vi "ni579x Validate LO Frequency.vi"(0 "Register Bus":refnum<class "ni579x Register Bus v1 Host.lvclass">=refnum, 1 "scope":string, 5 "frequency [Hz]":dbl format="%#_6p", 11 "Error In":errorcluster) -> (4 "Register Bus (out)":refnum<class "ni579x Register Bus v1 Host.lvclass">, 6 "coerced frequency [Hz]":dbl format="%#_6p", 15 "Error Out":errorcluster)   [LabVIEW 2015]
uses:
  <instrlib>/ni579x/Register Bus/v1/Host/ni579x Register Bus v1 Host.lvclass
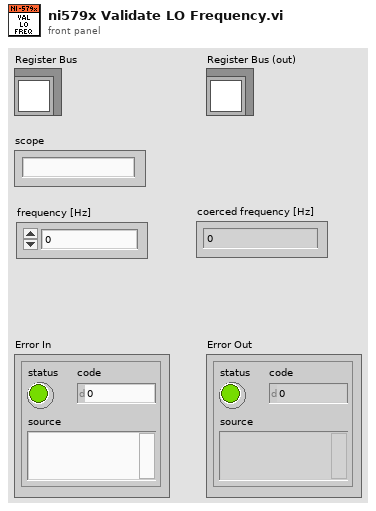
[diagram p1: front panel]
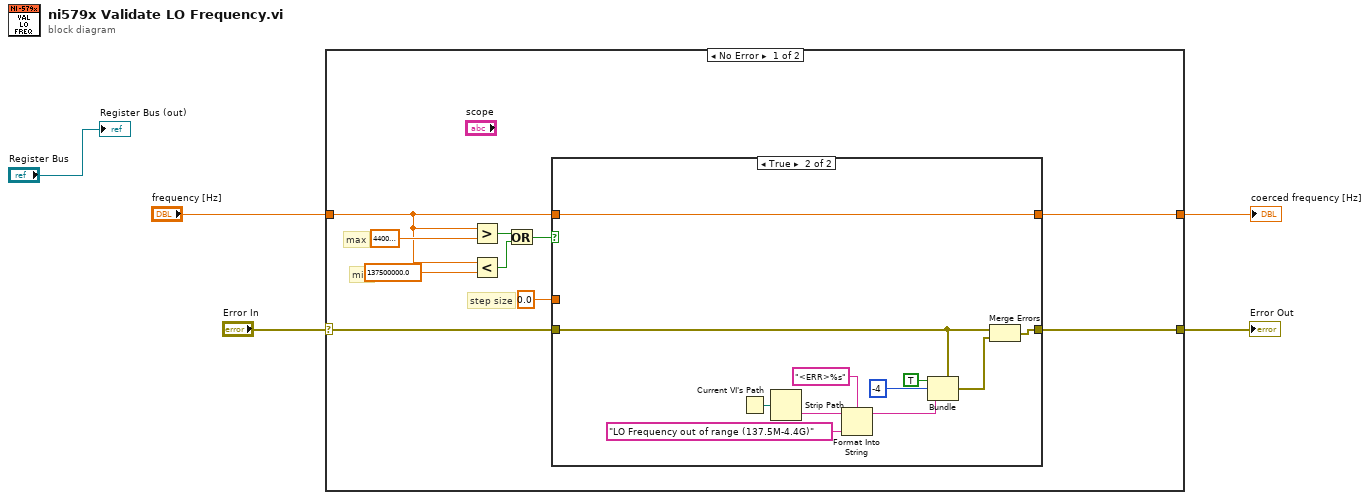
[diagram p0: block diagram]
diagram:
  n1 = case shown="No Error" "Error In" {
    selector: "Error In" -> [w8 w30]
    tunnel: [w6 w30] -> w4
    tunnel: "frequency [Hz]" -> [w10 w29]
    tunnel: [w7 w29] -> w1
    frame No Error {
      # "min"
      # "max"
      # "step size"
      n2 = Greater?(x=w10, y=4400000000.0) -> (0:w13:bool)
      n3 = Less?(x=w10, y=137500000.0) -> (x < y?=w12:bool)
      n4 = Or(x=w13, y=w12) -> (x .or. y?=w11:bool)
      n5 = case shown="True" w11 {
        tunnel: w10 -> [w16 w21]
        tunnel: 0.0 -> [_ _]
        tunnel: [w16 w21] -> w7
        tunnel: w8 -> [w17 w24]
        tunnel: [w17 w22] -> w6
        frame False {
        }
        frame True {
          n6 = Current VI's Path() -> (path=w27:path)
          n7 = Strip Path(path=w27) -> (name=w26:string)  [unwired: 1 out]
          n8 = Format Into String(format string="<ERR>%s", initial string=w26, "LO Frequency out of range (137.5M-4.4G)" ("input 1")) -> (resulting string=w25:string)  [unwired: 1 in, 1 out]
          n9 = Bundle(cluster=w24, "status"=TRUE, "code"=-4, "source"=w25) -> (w23:errorcluster)
          n10 = Merge Errors(w24, w23) -> (w22:errorcluster)
        }
      }
    }
    frame Error {
    }
  }
  "Error Out" <- w4
  "coerced frequency [Hz]" <- w1
  "Register Bus (out)" <- "Register Bus"
